vi "SignalProcessPT.vi"(4 "Volt Scale":dbl[](array[numeric]), 6 "PSI Scale":dbl[](array[numeric]), 7 "Enabled":bool, 8 "Warning High":dbl, 9 "Warning Low":dbl, 11 "Signal":dbl) -> (0 "Warning":bool, 1 "Disable":i32, 3 "Signal Out":dbl)   [LabVIEW 2016]
uses:
  <vilib>/gmath/NI_Gmath.lvlib
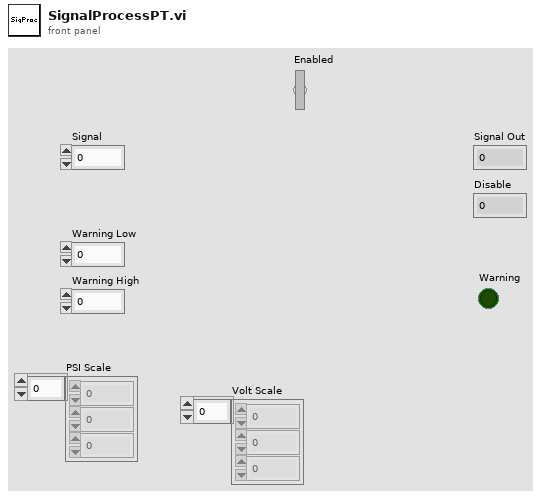
[diagram p1: front panel]
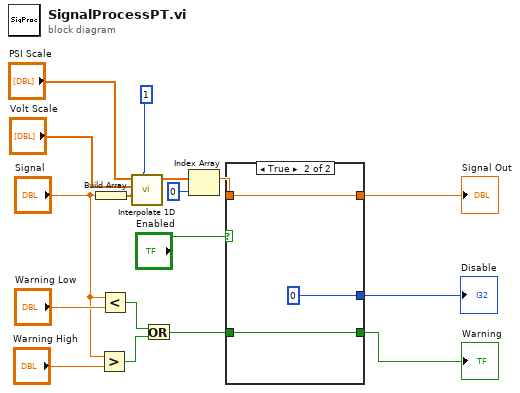
[diagram p0: block diagram]
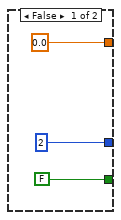
[diagram p2: hidden frame]
diagram:
  n1 = Build Array("Signal") -> (w4:dbl[])
  n2 = Greater?(x="Signal", y="Warning High") -> (0:w14:bool)
  n3 = Less?(x="Signal", y="Warning Low") -> (x < y?=w15:bool)
  n4 = call <vilib>:"Interpolate 1D.vi"("method"=1, "xi"=w4, "X"="Volt Scale", "Y"="PSI Scale") -> ("yi"=w7:dbl[])  [unwired: 5 in, 2 out]
  n5 = Or(x=w15, y=w14) -> (x .or. y?=w10:bool)
  n6 = Index Array(array=w7, index=0) -> (element=w3:dbl)
  n7 = case shown="True" "Enabled" {
    tunnel: [0.0 w23] -> w13
    tunnel: w3 -> [_ w23]
    tunnel: [2 0] -> w12
    tunnel: [FALSE w21] -> w11
    tunnel: w10 -> [_ w21]
    frame False {
    }
    frame True {
    }
  }
  "Signal Out" <- w13
  "Warning" <- w11
  "Disable" <- w12
